vi "HM8118 - Configure Measurement.vi"(6 "Manual Range (1:Range 1 and 25 Ohms)":u8(ring)=1 items=["Range 1 and 25 Ohms"=1, "Range 2 and 25 Ohms"=2, "Range 3 and 400 Ohms"=3, "Range 4 and 6.4 kOhms"=4, "Range 5 and 100kOhms"=5, "Range 6 and 100kOhms"=6], 7 "Circuit Type (2: Auto)":u16(ring)=2 items=["Series", "Parallel", "Auto"], 8 "error in (no error)":errorcluster, 9 "Auto Range (T: Enable)":bool=TRUE, 10 "Operation Mode (0: Auto)":u16(ring) items=["Auto", "L+Q", "L+R", "C+D", "C+R", "R+Q", "Z+Theta", "Y+Theta", "R+X", "G+B", "N+Theta", "M"], 11 "VISA resource name":refnum<visa-resource-name>) -> (0 "error out":errorcluster, 3 "VISA resource name out":refnum<visa-resource-name>)   [LabVIEW 2017]
doc: "Configures the parameter of operation, circuit type and range of the instrument."
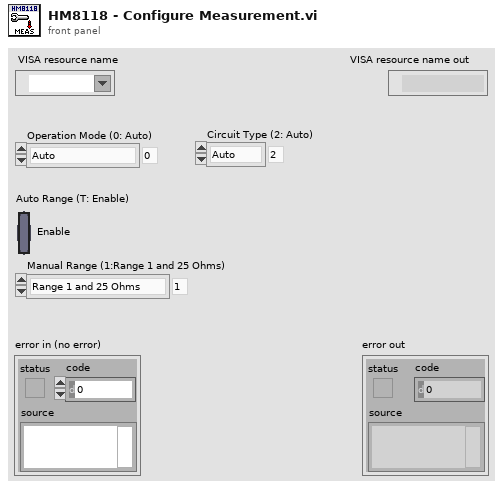
[diagram p1: front panel]
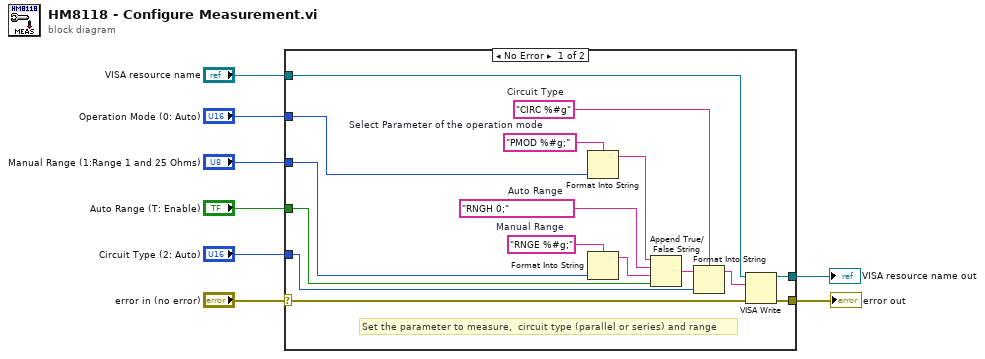
[diagram p0: block diagram]
diagram:
  n1 = case shown="No Error" "error in (no error)" {
    selector: "error in (no error)" -> [w9 w25]
    tunnel: "VISA resource name" -> [w24 w26]
    tunnel: "Auto Range (T: Enable)" -> [w20 _]
    tunnel: "Operation Mode (0: Auto)" -> [w18 _]
    tunnel: "Manual Range (1:Range 1 and 25 Ohms)" -> [w16 _]
    tunnel: "Circuit Type (2: Auto)" -> [w13 _]
    tunnel: [w11 w25] -> w3
    tunnel: [w10 w26] -> w2
    frame No Error {
      w15 = "CIRC %#g"  # Circuit Type
      w17 = "RNGH 0;"  # Auto Range
      w22 = "RNGE %#g;"  # Manual Range
      w23 = "PMOD %#g;"  # Select Parameter of the operation mode
      # "Set the parameter to measure,  circuit type (parallel or series) and range"
      n2 = Format Into String(format string=w23, w18) -> (resulting string=w19:string)  [unwired: 2 in, 1 out]
      n3 = Format Into String(format string=w22, w16) -> (resulting string=w21:string)  [unwired: 2 in, 1 out]
      n4 = Append True/False String(1:w20, 2:w21, 3:w17, 4:w19) -> (0:w14:string)
      n5 = Format Into String(format string=w15, initial string=w14, w13) -> (resulting string=w12:string)  [unwired: 1 in, 1 out]
      n6 = VISA Write(VISA resource name=w24, write buffer=w12, error in (no error)=w9) -> (VISA resource name out=w10:refnum<visa-resource-name>, error out=w11:errorcluster)  [unwired: 1 out]
    }
    frame Error {
    }
  }
  "error out" <- w3
  "VISA resource name out" <- w2
